vi "Clear maps and sessions.vi"(8 "error in":errorcluster, 11 "References":T1) -> (0 "error out":errorcluster)   [LabVIEW 2025, in "CAN-LIN Raw Bus Capture UI.lvlib"]
uses:
  CAN-LIN Raw Bus Capture UI.lvlib
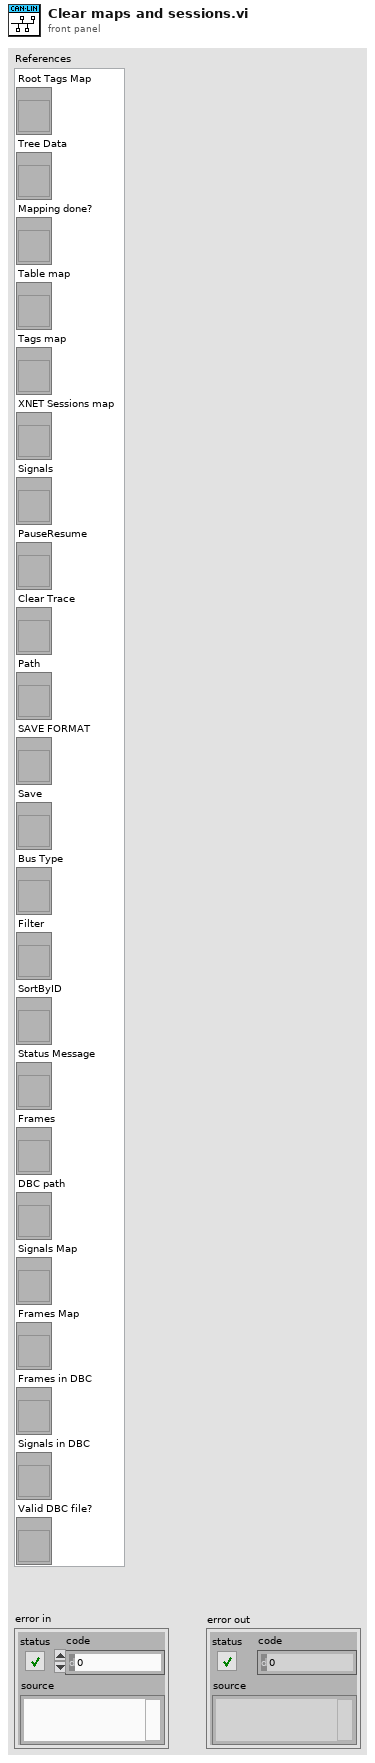
[diagram p1: front panel]
types:
  T1 = cluster{"Root Tags Map":refnum<vi>, "Tree Data":refnum<vi>, "Mapping done?":refnum<vi>, "Table map":refnum<vi>, "Tags map":refnum<vi>, "XNET Sessions map":refnum<vi>, "Signals":refnum<vi>, "PauseResume":refnum<vi>, "Clear Trace":refnum<vi>, "Path":refnum<vi>, "SAVE FORMAT":refnum<vi>, "Save":refnum<vi>, "Bus Type":refnum<vi>, "Filter":refnum<vi>, "SortByID":refnum<vi>, "Status Message":refnum<vi>, "Frames":refnum<vi>, "DBC path":refnum<vi>, "Signals Map":refnum<vi>, "Frames Map":refnum<vi>, "Frames in DBC":refnum<vi>, "Signals in DBC":refnum<vi>, "Valid DBC file?":refnum<vi>}
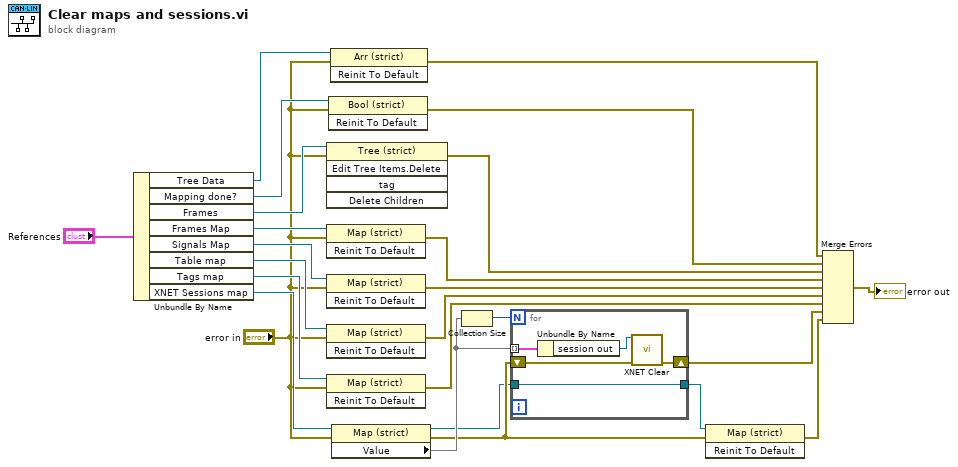
[diagram p0: block diagram]
diagram:
  n1 = Unbundle By Name("References") -> ("Tree Data"=w3:refnum<vi>, "Mapping done?"=w6:refnum<vi>, "Frames"=w20:refnum<vi>, "Frames Map"=w19:refnum<vi>, "Signals Map"=w18:refnum<vi>, "Table map"=w17:refnum<vi>, "Tags map"=w16:refnum<vi>, "XNET Sessions map"=w14:refnum<vi>)
  n2 = invoke on="Invoke Node" class="Tree (strict)" method="Edit Tree Items.Delete"(reference=w20, error in="error in") -> (error out=w22:errorcluster)  [unwired: 3 in, 4 out]
  n3 = invoke class="Map (strict)" method="Reinit To Default"(reference=w19, error in="error in") -> (error out=w21:errorcluster)  [unwired: 1 in, 2 out]
  n4 = invoke class="Map (strict)" method="Reinit To Default"(reference=w18, error in="error in") -> (error out=w9:errorcluster)  [unwired: 1 in, 2 out]
  n5 = invoke class="Map (strict)" method="Reinit To Default"(reference=w17, error in="error in") -> (error out=w10:errorcluster)  [unwired: 1 in, 2 out]
  n6 = invoke class="Map (strict)" method="Reinit To Default"(reference=w16, error in="error in") -> (error out=w15:errorcluster)  [unwired: 1 in, 2 out]
  n7 = invoke class="Bool (strict)" method="Reinit To Default"(reference=w6, error in="error in") -> (error out=w5:errorcluster)  [unwired: 1 in, 2 out]
  n8 = invoke class="Arr (strict)" method="Reinit To Default"(reference=w3, error in="error in") -> (error out=w2:errorcluster)  [unwired: 1 in, 2 out]
  n9 = property class="Map (strict)"(reference=w14, error in="error in") -> (reference out=w7:refnum<vi>, error out=w13:errorcluster, "Value"=w24:map{u32, refnum<k21>})
  n10 = Collection Size(1:w24) -> (0:w25:i32)
  n11 = for {
    N: w25 -> [_]
    tunnel: w24 -> [w30] mode=indexing
    shift-right: [w27] -> w11
    shift-left: w13 -> [w28]
    tunnel: [w26] -> w8
    tunnel: w7 -> [w26]
    n12 = Unbundle By Name(w30) -> ("session out"=w29:refnum<k21>)
    n13 = call <vilib>:"XNET Clear.vi"("session in"=w29, "error in (no error)"=w28) -> ("error out"=w27:errorcluster)  [unwired: 13 in]
  }
  n14 = invoke class="Map (strict)" method="Reinit To Default"(reference=w8, error in=w13) -> (error out=w12:errorcluster)  [unwired: 1 in, 2 out]
  n15 = Merge Errors(w2, w5, w22, w21, w9, w10, w15, w11, w12) -> (→"error out":errorcluster)
